vi "Generate Event.vi"(8 "Error In":errorcluster, 10 "Event":refnum<class "Event.lvclass">, 11 "Controller Actor In":refnum<class "Controller Actor.lvclass">) -> (0 "Error Out":errorcluster, 3 "Controller Actor Out":refnum<class "Controller Actor.lvclass">)   [LabVIEW 2016, in "Event Actors.lvlib" / "Controller Actor.lvclass"]
doc: "This method generates/fires the Event wired to the input. Firing an event looks up all actors who Registered to listen to this Event and sends to them this Event on a Zero Coupling based message defined during Registration. Errors on broadcasting the event i.e. enqueuer of the registrant not existing, are ignored.\n\n<b>IMPORTANT</b> - Only call this method within actor core of your Controller Actor. From helper loops call the Send Generate Event message to self. This is to make sure your actor works with all registered listeners."
uses:
  Controller Actor.lvclass
  Event/Event.lvclass
  Controller Actor.lvclass/Controller Actor.ctl
  Event Handler Details.ctl
  Event Handlers/Event Generated Msg/Event Generated Msg.lvclass
  C:/Program Files (x86)/National Instruments/LabVIEW 2016/vi.lib/ActorFramework/Message/Message.lvclass
  <vilib>/ActorFramework/Message Enqueuer/Message Enqueuer.lvclass
  Event Handlers/Event Generated Msg/Event Generated Msg.lvclass/Event Generated Msg.ctl
  <vilib>/ActorFramework/Message Enqueuer/Message Enqueuer.lvclass/Message Enqueuer.ctl
  <vilib>/ActorFramework/Message Enqueuer/Enqueue.vi
  <vilib>/ActorFramework/Message Priority Queue/Priority Enqueue.vi
  <resource>/AFDebug/Generate Trace for Message.vi
  <vilib>/Utility/LVClass/Get LV Class Name.vi
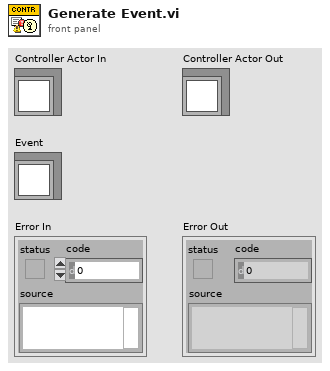
[diagram p1: front panel]
types:
  T1 = typedef "Event Actors.lvlib/Controller Actor.lvclass/Event Handler Details.ctl" = cluster{"Exclude From Broadcast":bool, "Paused":bool, "View Event Fire Handler":refnum<class "Event Generated Msg.lvclass">}
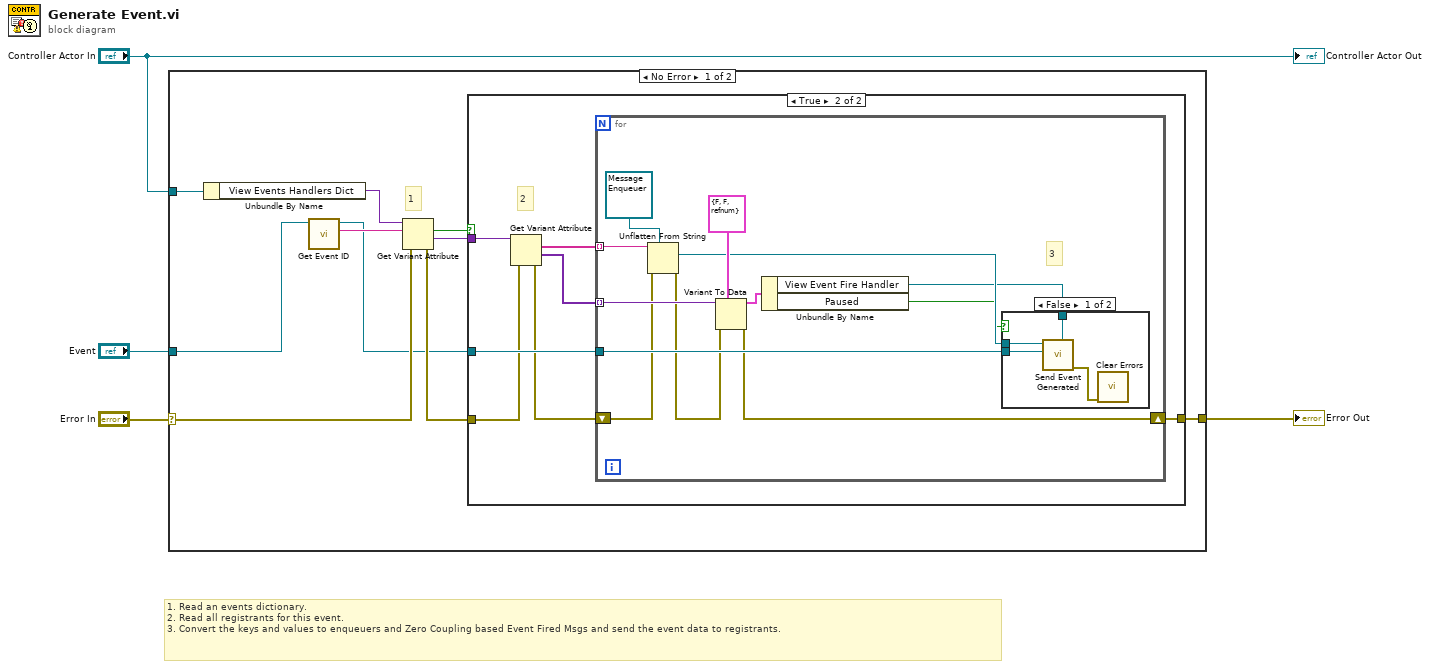
[diagram p0: block diagram]
diagram:
  # "1. Read an events dictionary.\n2. Read all registrants for this event.\n3. Convert the keys and values to enqueuers and Zero Coupling based Event Fired Msgs and send the event data to registrants."
  n1 = case shown="No Error" "Error In" {
    selector: "Error In" -> [w6 w39]
    tunnel: "Controller Actor In" -> [w14 _]
    tunnel: "Event" -> [w8 _]
    tunnel: [w13 w39] -> w2
    frame No Error {
      # "1"
      n2 = Unbundle By Name(w14) -> ("View Events Handlers Dict"=w12:variant)
      n3 = call-dynamic "Get Event ID.vi"("Event in"=w8) -> ("Event ID"=w7:string, "Event out"=w5:refnum<class "Event.lvclass">)  [unwired: 8 in, 1 out]
      n4 = Get Variant Attribute(Variant=w12, name=w7, error in=w6) -> (found=w9:bool, value=w10:variant, error out=w11:errorcluster)  [unwired: 1 in, 1 out]
      n5 = case shown="True" w9 {
        tunnel: w10 -> [_ w20]
        tunnel: w5 -> [_ w22]
        tunnel: w11 -> [w15 w17]
        tunnel: [w15 w21] -> w13
        frame False {
        }
        frame True {
          # "2"
          n6 = Get Variant Attribute(Variant=w20, error in=w17) -> (names=w19:string[], values=w18:variant[], error out=w16:errorcluster)  [unwired: 2 in, 1 out]
          n7 = for {
            tunnel: w19 -> [w26] mode=indexing
            tunnel: w18 -> [w34] mode=indexing
            tunnel: w22 -> [w32]
            shift-right: [w25] -> w21
            shift-left: w16 -> [w31]
            # "3"
            n8 = Unflatten From String(type=refnum<class "Message Enqueuer.lvclass"> refnum ("Message Enqueuer"), binary string=w26, error in (no error)=w31) -> (value=w27:refnum<class "Message Enqueuer.lvclass">, error out=w30:errorcluster)  [unwired: 2 in, 1 out]
            n9 = Variant To Data(error in=w30, type=T1 {"Exclude From Broadcast"=FALSE, "Paused"=FALSE, "View Event Fire Handler"=refnum} ("Message Type"), Variant=w34) -> (data=w33:T1, error out=w25:errorcluster)
            n10 = Unbundle By Name(w33) -> ("View Event Fire Handler"=w24:refnum<class "Event Generated Msg.lvclass">, "Paused"=w23:bool)
            n11 = case shown="False" w23 {
              tunnel: w24 -> [w38 _]
              tunnel: w32 -> [w37 _]
              tunnel: w27 -> [w35 _]
              frame False {
                n12 = call "Send Event Generated.vi"("Message Type"=w38, "Event Data"=w37, "Message Enqueuer"=w35) -> ("Error Out"=w36:errorcluster)  [unwired: 7 in, 1 out]
                n13 = call <vilib>:"Clear Errors.vi"("error in (no error)"=w36) -> ()  [unwired: 5 in, 2 out]
              }
              frame True {
              }
            }
          }
        }
      }
    }
    frame Error {
    }
  }
  "Error Out" <- w2
  "Controller Actor Out" <- "Controller Actor In"
